vi "CCE RRMA T030 SubVI03.vi"(10 "amp borde":u8=1, 11 "capa u8":u8[][](array[numeric])=array636x952[605472 elements]) -> (2 "phi":sgl[][](array[numeric]), 3 "new picture":picture)   [LabVIEW 2020]
doc: "Ceballos Conde Emanuel Rodríguez Ramírez Miguel Ángel 4MV6 Sistemas de visión artificial 2022/1\neste vi permite obtener el gradiente de una imagen asi como el angulo phi formade por el arco tangente de el gradiente en x e y de la imagen"
panel:
  # "Ceballos Conde Emanuel\nRodríguez Ramírez Miguel Ángel\n4MV6\nSistemas de visión artificial\n2022/1"
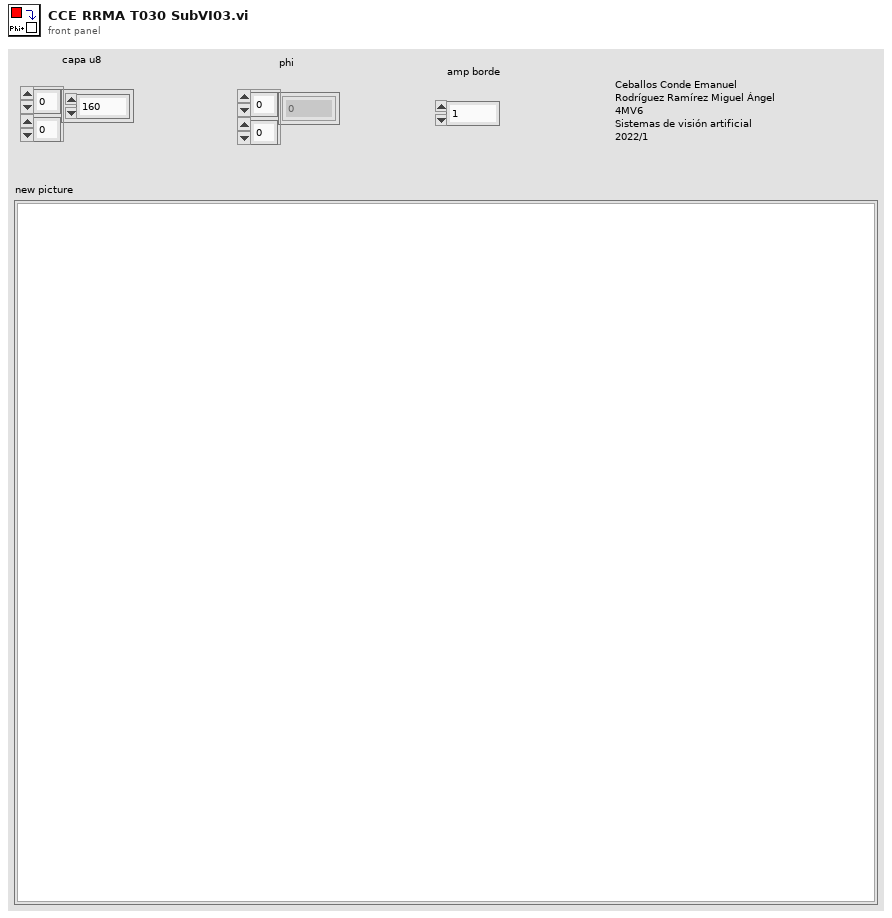
[diagram p1: front panel]
types:
  T1 = typedef "imagedata.ctl" = cluster{"image type":i32, "image depth":i32, "image":u8[], "mask":u8[], "colors":u32[], "Rectangle":cluster{"left":i16, "top":i16, "right":i16, "bottom":i16}}
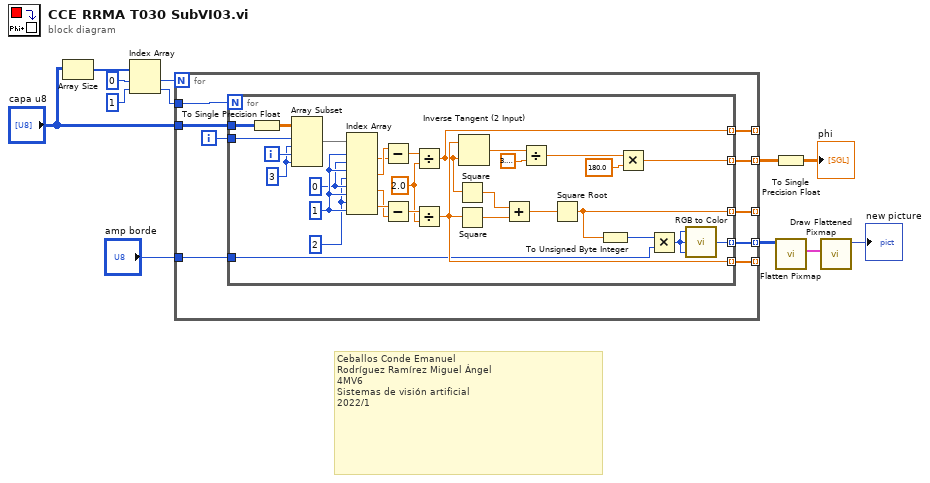
[diagram p0: block diagram]
diagram:
  # "Ceballos Conde Emanuel\nRodríguez Ramírez Miguel Ángel\n4MV6\nSistemas de visión artificial\n2022/1"
  n1 = Array Size(array="capa u8") -> (size(s)=w12:i32[])
  n2 = Index Array(array=w12, index #1=0 ("index"), index #2=1 ("index")) -> (element #1=w11:i32, element #2=w10:i32)
  n3 = for {
    N: w11 -> [_]
    tunnel: "capa u8" -> [w21]
    tunnel: w10 -> [w19]
    tunnel: [w18] -> _ mode=indexing
    tunnel: [w17] -> _ mode=indexing
    tunnel: [w16] -> _ mode=indexing
    tunnel: [w15] -> w3 mode=indexing
    tunnel: [w14] -> w7 mode=indexing
    tunnel: "amp borde" -> [w13]
    i -> [w20]
    n4 = for {
      N: w19 -> [_]
      tunnel: w21 -> [w52]
      tunnel: w20 -> [w50]
      tunnel: [w32] -> w18 mode=indexing
      tunnel: [w33] -> w17 mode=indexing
      tunnel: [w31] -> w16 mode=indexing
      tunnel: [w22] -> w15 mode=indexing
      tunnel: [w29] -> w14 mode=indexing
      tunnel: w13 -> [w27]
      i -> [w51]
      w38 = 2.0 ("y")
      w45 = 2 ("disabled index (col)")
      w46 = 0 ("disabled index (col)")
      w47 = 1 ("index (row)")
      w49 = 3 ("length")
      n5 = To Single Precision Float(number=w52) -> (single precision float=w37:sgl[][])
      n6 = Array Subset(array=w37, index (row)=w50, length (row)=w49, index (col)=w51, length (col)=w49) -> (w48:sgl[][])
      n7 = Index Array(array=w48, index (row) #1=w47, index (col) #1=w46, index (row) #2=w47, index (col) #2=w45, index (row) #3=w46, index (col) #3=w47, index (row) #4=w45, index (col) #4=w47) -> (element #1=w43:sgl, element #2=w44:sgl, element #3=w41:sgl, element #4=w42:sgl)
      n8 = Subtract(x=w44, y=w43) -> (x-y=w39:sgl)
      n9 = Subtract(x=w42, y=w41) -> (x-y=w40:sgl)
      n10 = Divide(x=w39, y=w38) -> (x/y=w32:dbl)
      n11 = Divide(x=w40, y=w38) -> (x/y=w33:dbl)
      n12 = Square(x=w32) -> (x^2=w35:dbl)
      n13 = Square(x=w33) -> (x^2=w34:dbl)
      n14 = Inverse Tangent (2 Input)(1:w32, 2:w33) -> (0:w26:dbl)
      n15 = Add(x=w35, y=w34) -> (x+y=w36:dbl)
      n16 = Divide(x=w26, y=3.141592653589793) -> (x/y=w24:dbl)
      n17 = Square Root(x=w36) -> (sqrt(x)=w31:dbl)
      n18 = To Unsigned Byte Integer(number=w31) -> (unsigned 8bit integer=w30:u8)
      n19 = Multiply(x=w24, y=180.0) -> (x*y=w22:dbl)
      n20 = Multiply(x=w30, y=w27) -> (x*y=w28:u8)
      n21 = call <vilib>:"RGB to Color.vi"("B"=w28, "G"=w28, "R"=w28) -> ("Color"=w29:u32)
    }
  }
  n22 = To Single Precision Float(number=w3) -> (single precision float=→"phi":sgl[][])
  n23 = call <vilib>:"Flatten Pixmap.vi"("24-bit pixmap"=w7) -> ("image data"=w6:T1)  [unwired: 10 in]
  n24 = call <vilib>:"Draw Flattened Pixmap.vi"("image data"=w6) -> ("new picture"=→"new picture":picture)  [unwired: 8 in]
